vi "Pre Launch Init.vi"(11 "Log in":refnum<class "Log.lvclass">) -> (0 "error out":errorcluster, 3 "Log out":refnum<class "Log.lvclass">)   [LabVIEW 2015, in "AMS UI.lvlib" / "Log.lvclass"]
doc: "(<B>Filename</B>: Actor Framework.lvlib:Actor.lvclass:Pre Launch Init.vi)\n\nDefines behavior that occurs after the Launch Actor method is invoked but before the actor's Actor Core method begins running.\n\nThe Pre Launch Init method is guaranteed to finish before the Launch Actor method returns to its caller and before the actor itself receives any messages. Any references that the Pre Launch Init method obtains are guaranteed to have the same lifetime as the actor itself. Any errors that the Pre Launch Init method returns will abort the launch.\n\nBy default, this method does nothing. A descendant class may override it to define behavior."
uses:
  Log.lvclass
  Log.lvclass/Log.ctl
  AMS Gas Actor/AMS Gas Actor.lvclass
  eActor Messages/Timeout Msg/Timeout Msg.lvclass
  <vilib>/ActorFramework/Message Enqueuer/Message Priority.ctl
  <vilib>/ActorFramework/Message Enqueuer/Message Enqueuer.lvclass
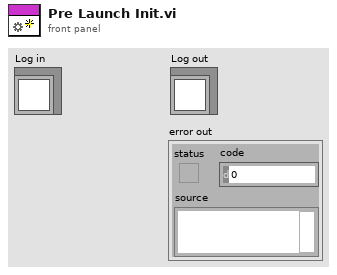
[diagram p1: front panel]
types:
  T1 = typedef "Actor Framework.lvlib/Message Enqueuer.lvclass/Message Priority.ctl" = enum16{"Low", "Normal", "High"}
  T2 = cluster{"Read Access":enum8{"Allowed", "Required", "None"}, "Write Access":enum8{"Allowed", "Required", "None"}}
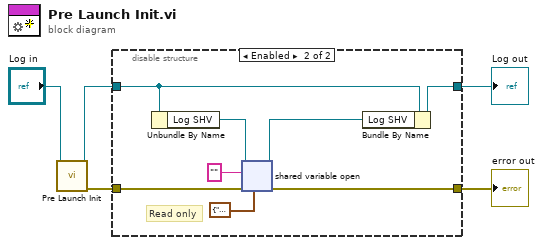
[diagram p0: block diagram]
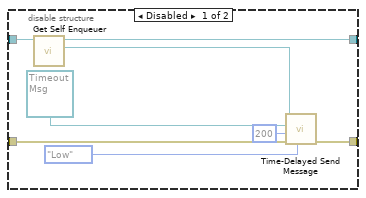
[diagram p2: hidden frame]
diagram:
  n1 = call-parent "Pre Launch Init.vi"("eActor in"="Log in") -> ("error out"=w2:errorcluster, "eActor out"=w4:refnum<class "Log.lvclass">)  [unwired: 9 in]
  n2 = disable-structure shown="Enabled" {
    disable-tunnel: w4 -> [w13 w21]
    disable-tunnel: [w12 w20] -> w3
    disable-tunnel: w2 -> [w11 w19]
    disable-tunnel: [w10 w18] -> w1
    frame Disabled {
      n3 = call-dynamic "Get Self Enqueuer.vi"("eActor in"=w13) -> ("Actor Framework:Message Enqueuer"=w9:refnum<class "Message Enqueuer.lvclass">, "eActor out"=w12:refnum<class "Log.lvclass">)  [unwired: 9 in]
      n4 = call <vilib>:"Time-Delayed Send Message.vi"("Message Priority (Normal)"=Message_Priority."Low", "error in (no error)"=w11, "Milliseconds To Wait"=200, "Message"=refnum<class "Timeout Msg.lvclass"> refnum ("Timeout Msg.lvclass"), "Message Enqueuer"=w9) -> ("error out"=w10:errorcluster)  [unwired: 5 in, 1 out]
    }
    frame Enabled {
      # "Read only"
      n5 = Unbundle By Name(w21) -> ("Log SHV"=w17:refnum<k21>)
      n6 = shared-variable-open(w17, w19, "", T2 {"Read Access"=enum."Allowed", "Write Access"=enum."None"} ("access")) -> (w16:refnum<k21>, w18:errorcluster)
      n7 = Bundle By Name(cluster=w21, "Log SHV"=w16) -> (w20:refnum<class "Log.lvclass">)
    }
  }
  "error out" <- w1
  "Log out" <- w3
